vi "BridgeComsData.vi"(8 "error in (no error)":errorcluster, 11 "connection ID in":refnum<k16>) -> (0 "error out":errorcluster, 1 "Buoy locations":cluster{"regular expression":string, i32, i32}[](array[cluster]), 2 "Tug GPS":cluster{"X pos":i32, "Y pos":i32, "Heading":dbl}, 3 "connection ID  out":refnum<k16>, 5 "GPS?":bool)   [LabVIEW 2014]
panel:
  out "UDP Time Out?":bool
  in  "Tug letter":string="G"
  # "This subVI  converts the UDP stream from the Tank Bridge into where your\ntugboat is and where the buoys are."
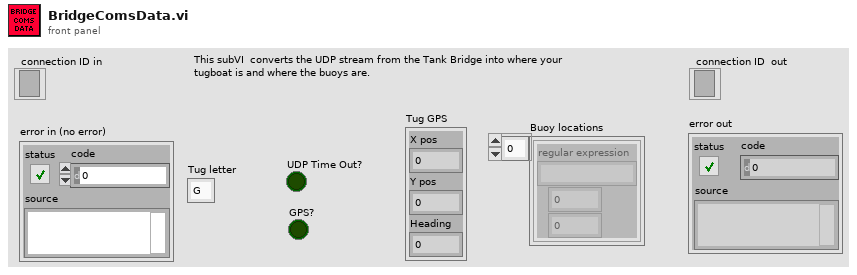
[diagram p1: front panel]
types:
  T1 = cluster{"regular expression":string, i32, i32, i32}
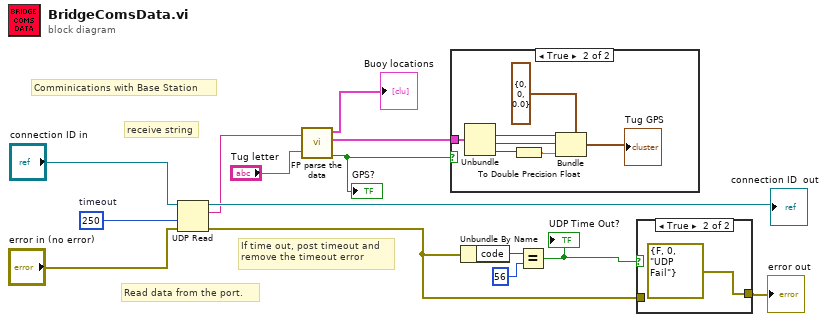
[diagram p0: block diagram]
diagram:
  w10 = 250  # timeout
  # "Comminications with Base Station"
  # "receive string"
  # "If time out, post timeout and\nremove the timeout error"
  # "Read data from the port."
  n1 = UDP Read(connection ID="connection ID in", timeout ms (25000)=w10, 8:"error in (no error)") -> (data out=w5:string, error out=w11:errorcluster, 3:→"connection ID  out":refnum<k16>)  [unwired: 1 in, 2 out]
  n2 = call "FP parse the data.vi"("Nav String"=w5, "Tug"="Tug letter") -> ("Buoy locations"=→"Buoy locations":cluster{"regular expression":string, i32, i32}[], "Tug Location"=w2:T1, "Valid?"=w1:bool)  [unwired: 1 out]
  "GPS?" <- w1
  n3 = case shown="True" w1 {
    tunnel: w2 -> [_ w21]
    frame False {
    }
    frame True {
      n4 = Unbundle(w21) -> (w20:i32, w19:i32, w17:i32)  [unwired: 1 out]
      n5 = To Double Precision Float(number=w17) -> (double precision float=w18:dbl)
      n6 = Bundle(cluster=cluster{"X pos":i32, "Y pos":i32, "Heading":dbl} {"X pos"=0, "Y pos"=0, "Heading"=0.0} ("Tug GPS"), "X pos"=w20, "Y pos"=w19, "Heading"=w18) -> (→"Tug GPS":cluster{"X pos":i32, "Y pos":i32, "Heading":dbl})
    }
  }
  n7 = Unbundle By Name(w11) -> ("code"=w14:i32)
  n8 = Equal?(x=w14, y=56) -> (x = y?=w12:bool)
  "UDP Time Out?" <- w12
  n9 = case shown="True" w12 {
    tunnel: [w22 errorcluster {"status"=FALSE, "code"=0, "source"="UDP Fail"} ("error out")] -> w7
    tunnel: w11 -> [w22 _]
    frame False {
    }
    frame True {
    }
  }
  "error out" <- w7
